vi "Dummy File Creator.vi"() -> ()   [LabVIEW 2019, in "Configuration File.lvlib" / "Configuration File.lvclass"]
uses:
  Configuration File.lvclass
panel:
  in  "Elevator Integers":cluster{"Key":string, "Numeric":u32}[](array[cluster])=[{"Key"="CAN Wrist", "Numeric"=6}, {"Key"="CAN Left Master", "Numeric"=13}, {"Key"="CAN Left Slave", "Numeric"=14}, {"Key"="CAN Right Master", "Numeric"=11}, {"Key"="CAN Right Slave", "Numeric"=12}, {"Key"="Arm Motion Magic Max Velocity", "Numeric"=1500}, {"Key"="Arm Motion Magic Max Acceleration", "Numeric"=1750}, {"Key"="Wrist Motion Magic Max Velocity", "Numeric"=22000}, {"Key"="Wrist Motion Magic Max Acceleration", "Numeric"=25000}]
  in  "Elevator Doubles":cluster{"Key":string, "Numeric":dbl}[](array[cluster])=[{"Key"="Elevator Arm P", "Numeric"=0.411027}, {"Key"="Elevator Arm I", "Numeric"=0.0}, {"Key"="Elevator Arm D", "Numeric"=0.0}, {"Key"="Elevator Arm F", "Numeric"=0.5708705357}, {"Key"="Elevator Wrist P", "Numeric"=0.02775}, {"Key"="Elevator Wrist I", "Numeric"=0.0}, {"Key"="Elevator Wrist D", "Numeric"=0.0}, {"Key"="Elevator Wrist F", "Numeric"=0.01515041059}]
  in  "Drive Booleans":cluster{"Key":string, "Boolean":bool}[](array[cluster])=[{"Key"="Sensor Right Invert", "Boolean"=TRUE}, {"Key"="Sensor Right Sensor Phase", "Boolean"=FALSE}, {"Key"="Sensor Left Invert", "Boolean"=FALSE}, {"Key"="Sensor Left Sensor Phase", "Boolean"=FALSE}]
  in  "Drive Doubles":cluster{"Key":string, "Numeric":dbl}[](array[cluster])=[{"Key"="Left Sensor Phase P", "Numeric"=0.08}, {"Key"="Left Sensor Phase I", "Numeric"=0.0}, {"Key"="Left Sensor Phase D", "Numeric"=0.0}, {"Key"="Left Sensor Phase F", "Numeric"=0.0682}, {"Key"="Velocity High Gear P", "Numeric"=0.04}, {"Key"="Velocity High Gear I", "Numeric"=0.0}, {"Key"="Velocity High Gear D", "Numeric"=0.0}, {"Key"="Velocity High Gear F", "Numeric"=0.0341}, {"Key"="Motion Magic Primary Low Gear P", "Numeric"=0.08}, {"Key"="Motion Magic Primary Low Gear I", "Numeric"=0.0}, {"Key"="Motion Magic Primary Low Gear D", "Numeric"=0.0}, {"Key"="Motion Magic Primary Low Gear F", "Numeric"=0.0341}, {"Key"="Motion Magic Primary High Gear P", "Numeric"=0.04}, {"Key"="Motion Magic Primary High Gear I", "Numeric"=0.0}, {"Key"="Motion Magic Primary High Gear D", "Numeric"=0.0}, {"Key"="Motion Magic Primary High Gear F", "Numeric"=0.01705}, {"Key"="Motion Magic Secondary Low Gear P", "Numeric"=0.007}, {"Key"="Motion Magic Secondary Low Gear I", "Numeric"=0.0}, {"Key"="Motion Magic Secondary Low Gear D", "Numeric"=0.0}, {"Key"="Motion Magic Secondary Low Gear F", "Numeric"=0.0}, {"Key"="Motion Magic Secondary High Gear P", "Numeric"=0.0035}, {"Key"="Motion Magic Secondary High Gear I", "Numeric"=0.0}, {"Key"="Motion Magic Secondary High Gear D", "Numeric"=0.0}, {"Key"="Motion Magic Secondary High Gear F", "Numeric"=0.0}]
  in  "Drive Integers":cluster{"Key":string, "Numeric":u32}[](array[cluster])=[{"Key"="CAN LeftPod Talon", "Numeric"=27}, {"Key"="CAN LeftPod Victor1", "Numeric"=28}, {"Key"="CAN LeftPod Victor2", "Numeric"=29}, {"Key"="CAN RightPod Talon", "Numeric"=30}, {"Key"="CAN RightPod Victor1", "Numeric"=31}, {"Key"="CAN RightPod Victor2", "Numeric"=32}, {"Key"="CAN Pigeon", "Numeric"=1}, {"Key"="Low Gear Max Velocity", "Numeric"=15000}, {"Key"="High Gear Max Velocity", "Numeric"=30000}, {"Key"="Motion Magic Low Gear Max Velocity", "Numeric"=30000}, {"Key"="Motion Magic Low Gear Max Acceleration", "Numeric"=30000}, {"Key"="Motion Magic High Gear Max Velocity", "Numeric"=60000}, {"Key"="Motion Magic High Gear Max Acceleration", "Numeric"=60000}]
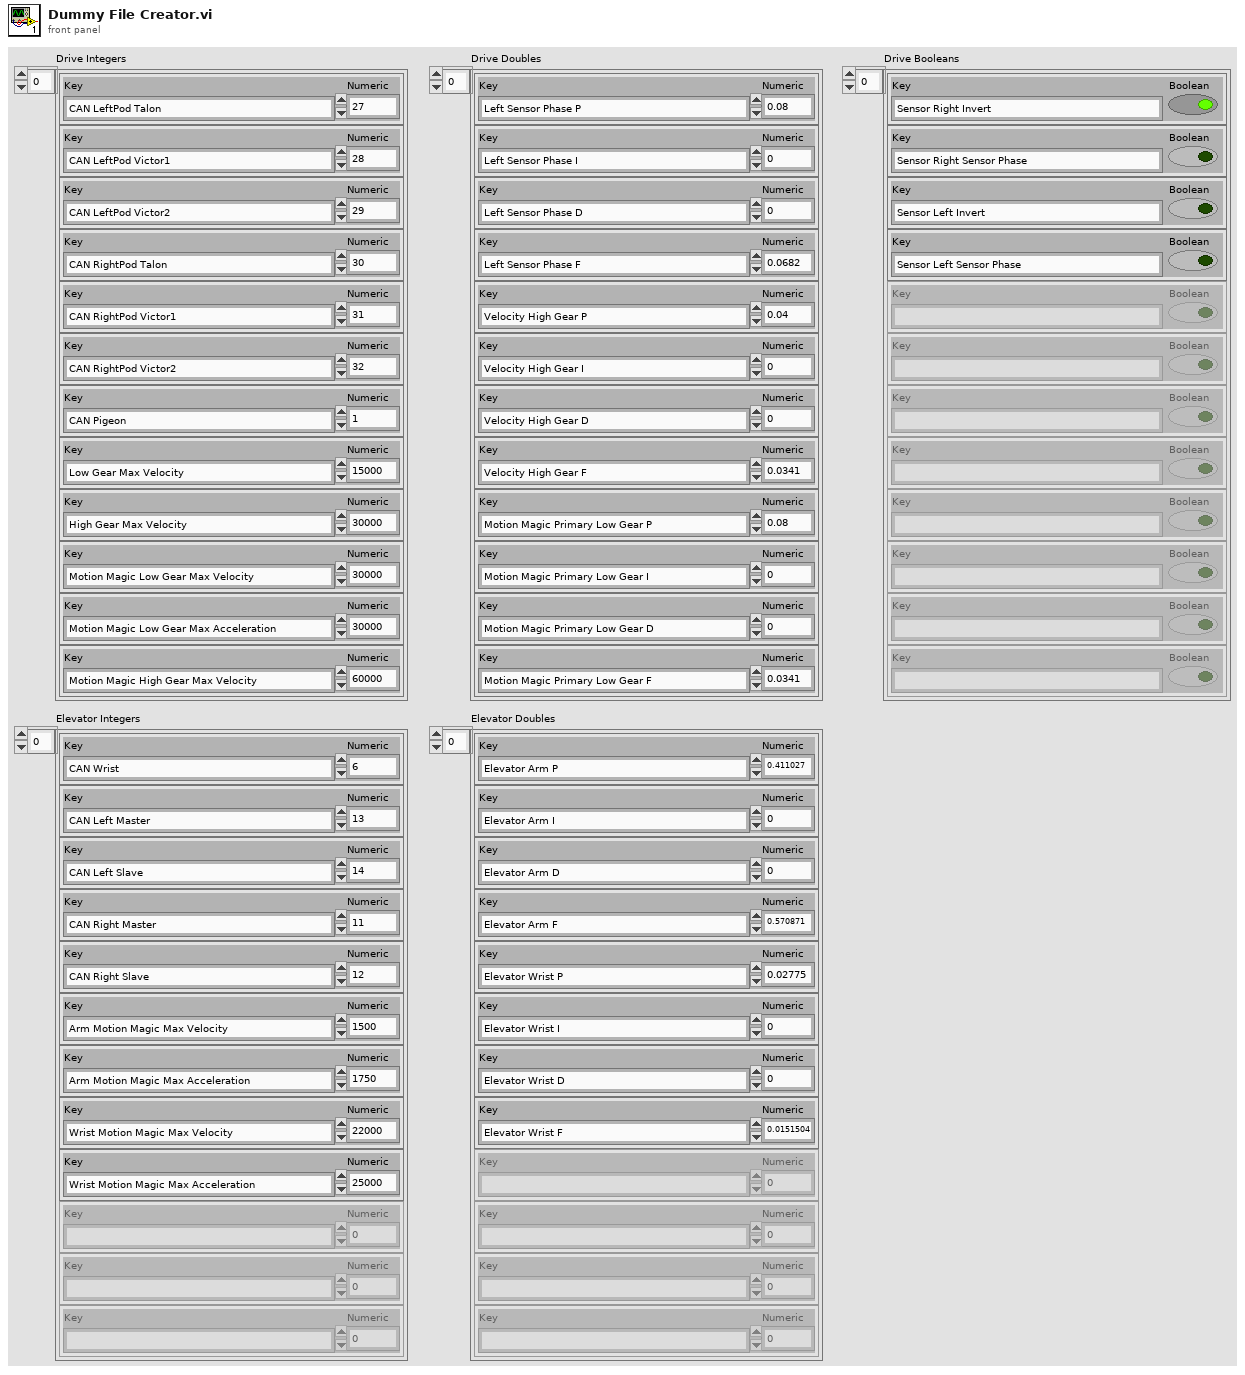
[diagram p1: front panel]
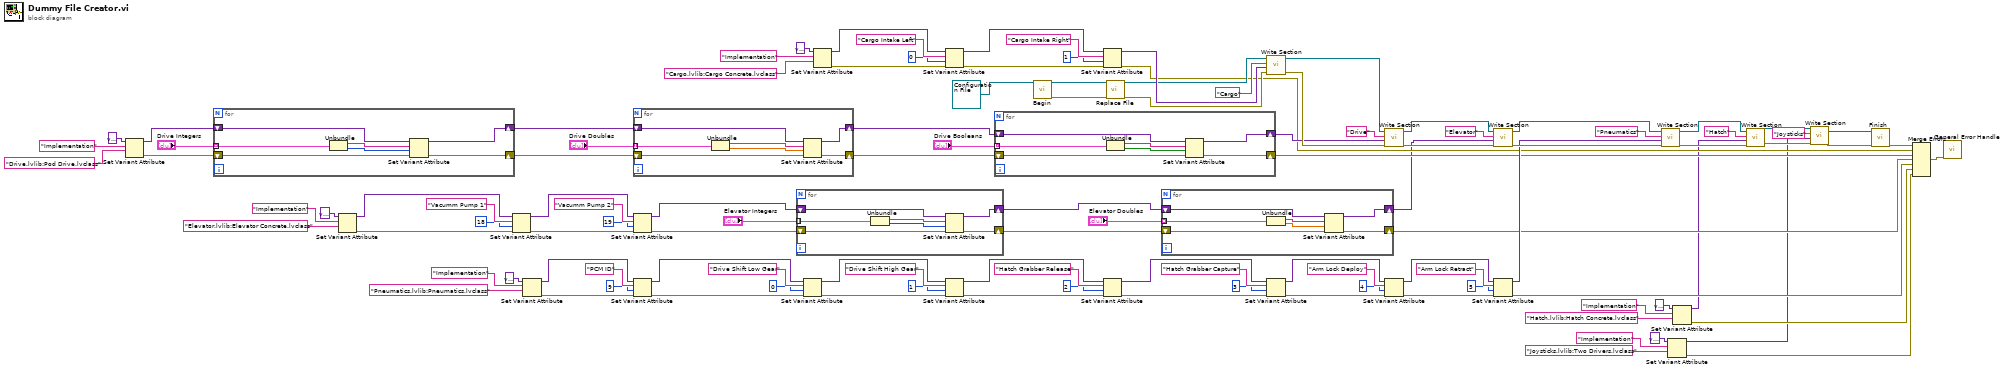
[diagram p0: block diagram]
diagram:
  n1 = Set Variant Attribute(Variant=variant, name="Implementation", value="Drive.lvlib:Pod Drive.lvclass" ("name")) -> (Variant out=w82:variant, error out=w68:errorcluster)  [unwired: 1 in, 1 out]
  n2 = for {
    shift-right: [w120] -> w42
    shift-left: w82 -> [w121]
    shift-right: [w118] -> w41
    shift-left: w68 -> [w119]
    tunnel: "Drive Integers" -> [w117] mode=indexing
    n3 = Unbundle(w117) -> ("Key"=w116:string, "Numeric"=w115:u32)
    n4 = Set Variant Attribute(Variant=w121, name=w116, value=w115, error in=w119) -> (Variant out=w120:variant, error out=w118:errorcluster)  [unwired: 1 out]
  }
  n5 = Set Variant Attribute(Variant=variant, name="Implementation", value="Elevator.lvlib:Elevator Concrete.lvclass" ("name")) -> (Variant out=w81:variant, error out=w69:errorcluster)  [unwired: 1 in, 1 out]
  n6 = Set Variant Attribute(Variant=w81, name="Vacumm Pump 1", value=u8 18, error in=w69) -> (Variant out=w79:variant, error out=w46:errorcluster)  [unwired: 1 out]
  n7 = Set Variant Attribute(Variant=variant, name="Implementation", value="Pneumatics.lvlib:Pneumatics.lvclass" ("name")) -> (Variant out=w80:variant, error out=w70:errorcluster)  [unwired: 1 in, 1 out]
  n8 = for {
    shift-right: [w127] -> w38
    shift-left: w42 -> [w128]
    shift-right: [w125] -> w39
    shift-left: w41 -> [w126]
    tunnel: "Drive Doubles" -> [w124] mode=indexing
    n9 = Unbundle(w124) -> ("Key"=w123:string, "Numeric"=w122:dbl)
    n10 = Set Variant Attribute(Variant=w128, name=w123, value=w122, error in=w126) -> (Variant out=w127:variant, error out=w125:errorcluster)  [unwired: 1 out]
  }
  n11 = Set Variant Attribute(Variant=w79, name="Vacumm Pump 2", value=u8 19, error in=w46) -> (Variant out=w22:variant, error out=w21:errorcluster)  [unwired: 1 out]
  n12 = Set Variant Attribute(Variant=w80, name="PCM ID", value=u8 9, error in=w70) -> (Variant out=w78:variant, error out=w77:errorcluster)  [unwired: 1 out]
  n13 = for {
    shift-right: [w134] -> w24
    shift-left: w22 -> [w135]
    shift-right: [w132] -> w25
    shift-left: w21 -> [w133]
    tunnel: "Elevator Integers" -> [w131] mode=indexing
    n14 = Unbundle(w131) -> ("Key"=w130:string, "Numeric"=w129:u32)
    n15 = Set Variant Attribute(Variant=w135, name=w130, value=w129, error in=w133) -> (Variant out=w134:variant, error out=w132:errorcluster)  [unwired: 1 out]
  }
  n16 = Set Variant Attribute(Variant=w78, name="Drive Shift Low Gear", value=u8 0, error in=w77) -> (Variant out=w76:variant, error out=w75:errorcluster)  [unwired: 1 out]
  n17 = Set Variant Attribute(Variant=variant, name="Implementation", value="Cargo.lvlib:Cargo Concrete.lvclass" ("name")) -> (Variant out=w113:variant, error out=w112:errorcluster)  [unwired: 1 in, 1 out]
  n18 = Set Variant Attribute(Variant=w113, name="Cargo Intake Left", value=u8 0, error in=w112) -> (Variant out=w111:variant, error out=w110:errorcluster)  [unwired: 1 out]
  n19 = Set Variant Attribute(Variant=w76, name="Drive Shift High Gear", value=u8 1, error in=w75) -> (Variant out=w74:variant, error out=w73:errorcluster)  [unwired: 1 out]
  n20 = for {
    shift-right: [w141] -> w37
    shift-left: w38 -> [w142]
    shift-right: [w139] -> w29
    shift-left: w39 -> [w140]
    tunnel: "Drive Booleans" -> [w138] mode=indexing
    n21 = Unbundle(w138) -> ("Key"=w137:string, "Boolean"=w136:bool)
    n22 = Set Variant Attribute(Variant=w142, name=w137, value=w136, error in=w140) -> (Variant out=w141:variant, error out=w139:errorcluster)  [unwired: 1 out]
  }
  n23 = call-dynamic "Begin.vi"("Configuration File in"=refnum<class "Configuration File.lvclass"> refnum) -> ("error out"=w34:errorcluster, "Configuration File out"=w35:refnum<class "Configuration File.lvclass">)  [unwired: 9 in]
  n24 = Set Variant Attribute(Variant=w111, name="Cargo Intake Right", value=u8 1, error in=w110) -> (Variant out=w108:variant, error out=w30:errorcluster)  [unwired: 1 out]
  n25 = Set Variant Attribute(Variant=w74, name="Hatch Grabber Release", value=u8 2, error in=w73) -> (Variant out=w72:variant, error out=w71:errorcluster)  [unwired: 1 out]
  n26 = call "Replace File.vi"("error in (no error)"=w34, "Configuration File in"=w35) -> ("error out"=w32:errorcluster, "Configuration File out"=w33:refnum<class "Configuration File.lvclass">)  [unwired: 8 in]
  n27 = for {
    shift-right: [w148] -> w2
    shift-left: w24 -> [w149]
    shift-right: [w146] -> w20
    shift-left: w25 -> [w147]
    tunnel: "Elevator Doubles" -> [w145] mode=indexing
    n28 = Unbundle(w145) -> ("Key"=w144:string, "Numeric"=w143:dbl)
    n29 = Set Variant Attribute(Variant=w149, name=w144, value=w143, error in=w147) -> (Variant out=w148:variant, error out=w146:errorcluster)  [unwired: 1 out]
  }
  n30 = call-dynamic "Write Section.vi"("error in (no error)"=w32, "Section Data"=w108, "Section Name"="Cargo", "Configuration File in"=w33) -> ("error out"=w99:errorcluster, "Configuration File out"=w100:refnum<class "Configuration File.lvclass">)  [unwired: 6 in]
  n31 = Set Variant Attribute(Variant=w72, name="Hatch Grabber Capture", value=u8 3, error in=w71) -> (Variant out=w61:variant, error out=w60:errorcluster)  [unwired: 1 out]
  n32 = call-dynamic "Write Section.vi"("error in (no error)"=w99, "Section Data"=w37, "Section Name"="Drive", "Configuration File in"=w100) -> ("error out"=w97:errorcluster, "Configuration File out"=w98:refnum<class "Configuration File.lvclass">)  [unwired: 6 in]
  n33 = Set Variant Attribute(Variant=w61, name="Arm Lock Deploy", value=u8 4, error in=w60) -> (Variant out=w59:variant, error out=w62:errorcluster)  [unwired: 1 out]
  n34 = call-dynamic "Write Section.vi"("error in (no error)"=w97, "Section Data"=w2, "Section Name"="Elevator", "Configuration File in"=w98) -> ("error out"=w95:errorcluster, "Configuration File out"=w96:refnum<class "Configuration File.lvclass">)  [unwired: 6 in]
  n35 = Set Variant Attribute(Variant=w59, name="Arm Lock Retract", value=u8 5, error in=w62) -> (Variant out=w56:variant, error out=w28:errorcluster)  [unwired: 1 out]
  n36 = call-dynamic "Write Section.vi"("error in (no error)"=w95, "Section Data"=w56, "Section Name"="Pneumatics", "Configuration File in"=w96) -> ("error out"=w17:errorcluster, "Configuration File out"=w18:refnum<class "Configuration File.lvclass">)  [unwired: 6 in]
  n37 = Set Variant Attribute(Variant=variant, name="Implementation", value="Joysticks.lvlib:Two Drivers.lvclass" ("name")) -> (Variant out=w3:variant, error out=w4:errorcluster)  [unwired: 1 in, 1 out]
  n38 = Set Variant Attribute(Variant=variant, name="Implementation", value="Hatch.lvlib:Hatch Concrete.lvclass" ("name")) -> (Variant out=w13:variant, error out=w12:errorcluster)  [unwired: 1 in, 1 out]
  n39 = call-dynamic "Write Section.vi"("error in (no error)"=w17, "Section Data"=w13, "Section Name"="Hatch", "Configuration File in"=w18) -> ("error out"=w10:errorcluster, "Configuration File out"=w11:refnum<class "Configuration File.lvclass">)  [unwired: 6 in]
  n40 = call-dynamic "Write Section.vi"("error in (no error)"=w10, "Section Data"=w3, "Section Name"="Joysticks", "Configuration File in"=w11) -> ("error out"=w8:errorcluster, "Configuration File out"=w9:refnum<class "Configuration File.lvclass">)  [unwired: 6 in]
  n41 = call-dynamic "Finish.vi"("error in (no error)"=w8, "Configuration File in"=w9) -> ("error out"=w31:errorcluster)  [unwired: 6 in, 3 out]
  n42 = Merge Errors(w31, w30, w29, w20, w28, w12, w4) -> (w27:errorcluster)
  n43 = call <vilib>:"General Error Handler.vi"("error in (no error)"=w27) -> ()  [unwired: 10 in, 5 out]
